vi "SOM.vi"(8 "Stopp":bool, 10 "SLOT":i32=100, 11 "USB":i32) -> ()   [LabVIEW 2020]
doc: "This VI provides a GUI for SOM modules. It implements an abstract module interface, where callers provide the only necessary and sufficient information for callee modules via the datafields USB, SLOT and Stopp. All module intern information are handled hidden by the module. Thereby, a caller must not \"know\" about such internals."
panel:
  in  "BurstDat[i]":T1={"[i]"=1, "BurstLen[i]"=1, "SyncEna[i]"=TRUE, "OutpEna[i]"=TRUE} {"BurstLen[i]" min=0 max=16777215 step=1}
  in  "Burst Data":T2(array[cluster]) {"BurstLen[i]" min=0 max=16777215 step=1}
  in  "AUX In Ctrl":u8(ring) items=["free running", "running if AUX IN is on High", "running if AUX IN is on Low"]
  in  "AUX Out Ctrl":u8(ring) items=["disabled", "enabled"]
  in  "Sync Enable":bool[](array[boolean])=[TRUE, FALSE, FALSE, TRUE, FALSE, FALSE, FALSE, FALSE]
  in  "Burst Out":bool[](array[boolean])=[TRUE, TRUE, FALSE, FALSE, TRUE, FALSE, FALSE, FALSE]
  in  "TriggerLevel [mV]":i32=421 min=-1200 max=1200 step=100 format="%5d"
  in  "Burst Length":i32[](array[numeric])=[1, 0, 2, 0, 0, 0, 0, 0]
  in  "Invert":bool=TRUE
  in  "Syncmask":u8
  in  "Presync":u8=4
  in  "Divider":u8=80
  in  "Base Osc./Trigger":i32(ring)=2
  # "Idx   Burst Length       Sync Enable       Out Enable"
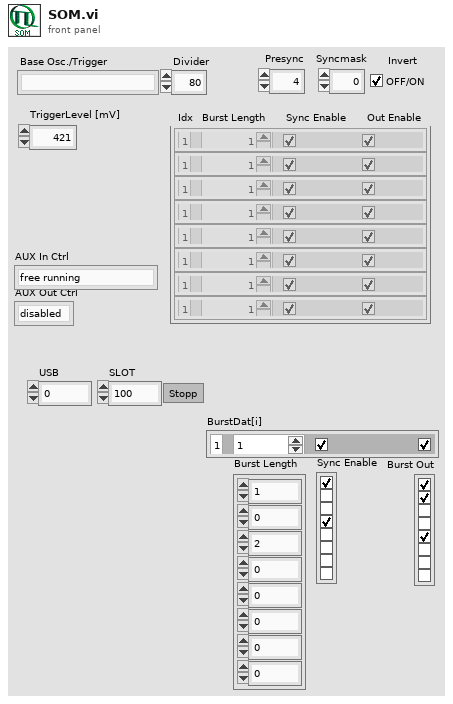
[diagram p1: front panel]
types:
  T1 = cluster{"[i]":i32, "BurstLen[i]":i32, "SyncEna[i]":bool, "OutpEna[i]":bool}
  T2 = cluster{"[i]":i32, "BurstLen[i]":i32, "SyncEna[i]":bool, "OutpEna[i]":bool}[]
  T3 = cluster{"Divider":u8, "PreSync":u8, "MaskSync":u8}
  T4 = cluster{"OutEnable":u8, "SyncEnable":u8, "SyncInverse":enum8{"Standard_Sync_Mask", "Inverse_Sync_Mask"}}
  T5 = cluster{"Divider":u8, "PreSync":u8, "SyncMask":u8}
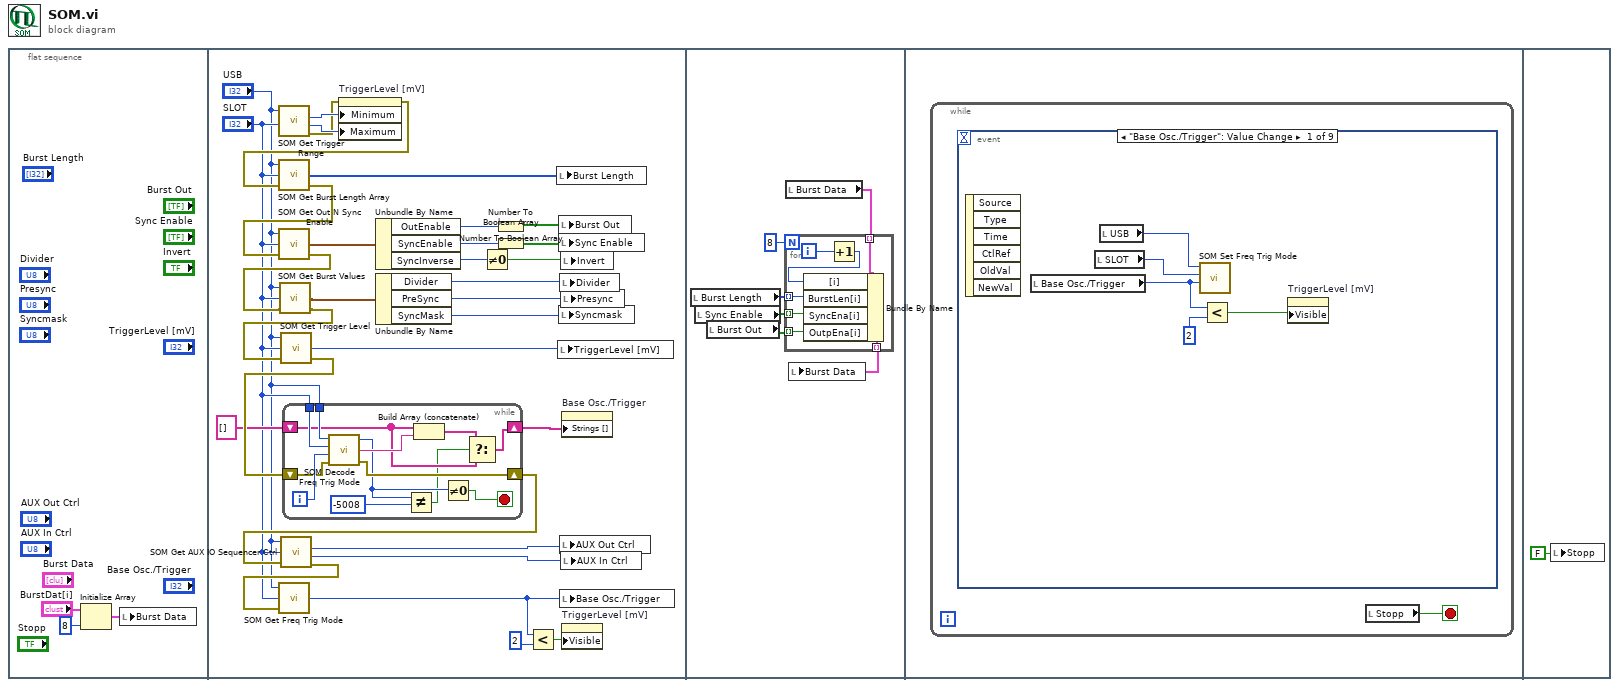
[diagram p0: block diagram]
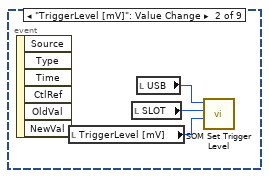
[diagram p2: hidden frame]
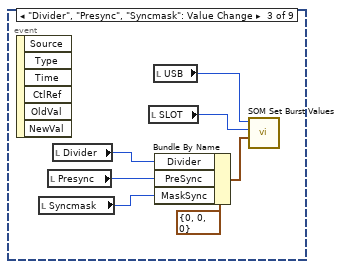
[diagram p3: hidden frame]
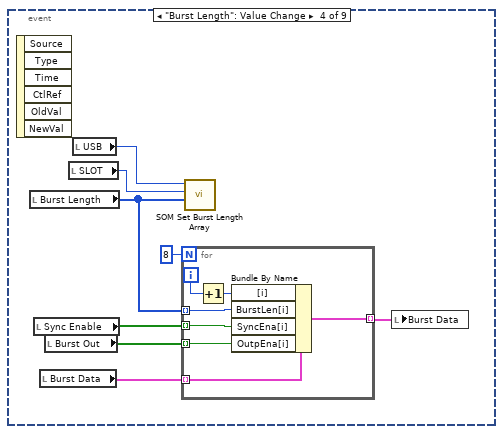
[diagram p4: hidden frame]
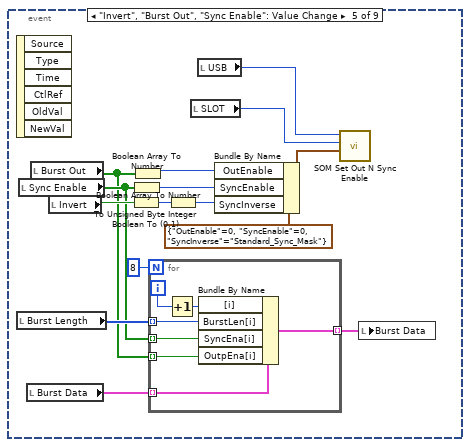
[diagram p5: hidden frame]
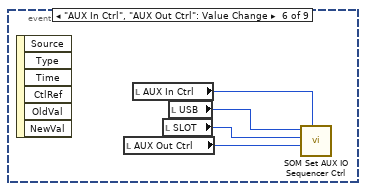
[diagram p6: hidden frame]
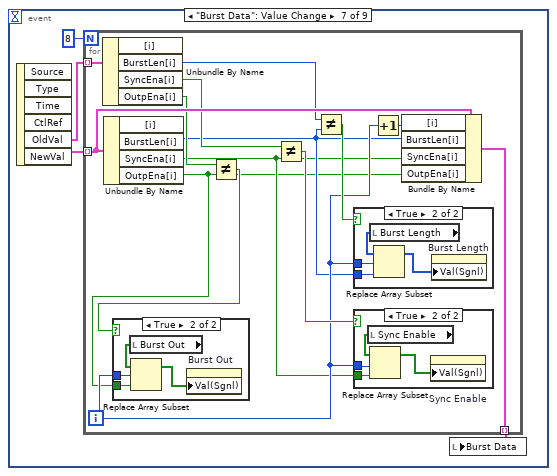
[diagram p7: hidden frame]
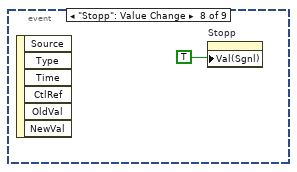
[diagram p11: hidden frame]
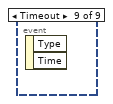
[diagram p12: hidden frame]
diagram:
  n1 = flat-sequence {
    frame #0 {
      n2 = Initialize Array("BurstDat[i]", 8 ("dimension size")) -> (w3:T2)
      n3 = local write "Burst Data"(w3) -> ()
    }
    frame #1 {
      n4 = call "SOM Get Trigger Range.vi"("DevIdx"="USB", "SlotId"="SLOT") -> ("MilliVoltLow"=w35:i32, "MilliVoltHigh"=w34:i32, "error out"=w33:errorcluster)  [unwired: 1 in, 1 out]
      n5 = property on="TriggerLevel [mV]" class="DigNum (strict)"(error in=w33, "Minimum"=w35, "Maximum"=w34) -> (error out=w32:errorcluster)  [unwired: 1 in, 1 out]
      n6 = call "SOM Get Burst Length Array.vi"("error in (no error)"=w32, "SlotId"="SLOT", "DevIdx"="USB") -> ("error out"=w12:errorcluster, "SOM Burst Length Array"=w5:i32[])  [unwired: 1 out]
      n7 = call "SOM Get Out N Sync Enable.vi"("error in (no error)"=w12, "SlotId"="SLOT", "DevIdx"="USB") -> ("error out"=w9:errorcluster, "SOM Out N Sync Enable"=w11:T4)  [unwired: 1 out]
      n8 = call "SOM Get Burst Values.vi"("error in (no error)"=w9, "SlotId"="SLOT", "DevIdx"="USB") -> ("error out"=w10:errorcluster, "SOM Burst Values"=w8:T5)  [unwired: 1 out]
      n9 = call "SOM Get Trigger Level.vi"("error in (no error)"=w10, "SlotId"="SLOT", "DevIdx"="USB") -> ("error out"=w21:errorcluster, "MilliVolt"=w22:i32)  [unwired: 1 out]
      n10 = while {
        tunnel: "USB" -> [w47]
        tunnel: "SLOT" -> [w46]
        shift-right: [w44] -> w15
        shift-left: w21 -> [w43]
        shift-right: [w39] -> w19
        shift-left: string[] [] -> [w37]
        i -> [w48]
        stop <- w45 stop-if-true
        n11 = call "SOM Decode Freq Trig Mode.vi"("error in (no error)"=w43, "FreqTrigMode"=w48, "SlotId"=w46, "DevIdx"=w47) -> ("error out"=w44:errorcluster, "FreqTrigMode"=w42:string, "function return"=w41:i32)
        n12 = Not Equal?(x=w41, y=-5008) -> (x != y?=w36:bool)
        n13 = Build Array (concatenate)(w37, w42) -> (w38:string[])
        n14 = Not Equal To 0?(x=w41) -> (x != 0?=w45:bool)
        n15 = Select(t=w38, s=w36, f=w37) -> (s? t:f=w39:string[])
      }
      n16 = call "SOM Get AUX IO Sequencer Ctrl.vi"("DevIdx"="USB", "SlotId"="SLOT", "error in (no error)"=w15) -> ("AUX Out Ctrl"=w4:u8, "AUX In Ctrl"=w13:u8, "error out"=w14:errorcluster)  [unwired: 1 out]
      n17 = call "SOM Get Freq Trig Mode.vi"("error in (no error)"=w14, "SlotId"="SLOT", "DevIdx"="USB") -> ("FreqTrigMode"=w16:i32)  [unwired: 2 out]
      n18 = Unbundle By Name(w11) -> ("OutEnable"=w31:u8, "SyncEnable"=w29:u8, "SyncInverse"=w27:enum8{"Standard_Sync_Mask", "Inverse_Sync_Mask"})
      n19 = Unbundle By Name(w8) -> ("Divider"=w23:u8, "PreSync"=w24:u8, "SyncMask"=w25:u8)
      n20 = Not Equal To 0?(x=w27) -> (x != 0?=w26:bool)
      n21 = Number To Boolean Array(number=w31) -> (Boolean array=w30:bool[])
      n22 = Number To Boolean Array(number=w29) -> (Boolean array=w28:bool[])
      n23 = Less?(x=w16, y=2) -> (x < y?=w18:bool)
      n24 = local write "Burst Length"(w5) -> ()
      n25 = local write "TriggerLevel [mV]"(w22) -> ()
      n26 = local write "Burst Out"(w30) -> ()
      n27 = local write "Sync Enable"(w28) -> ()
      n28 = local write "Syncmask"(w25) -> ()
      n29 = local write "Divider"(w23) -> ()
      n30 = local write "AUX Out Ctrl"(w4) -> ()
      n31 = local write "Base Osc./Trigger"(w16) -> ()
      n32 = local write "Invert"(w26) -> ()
      n33 = local write "Presync"(w24) -> ()
      n34 = local write "AUX In Ctrl"(w13) -> ()
      n35 = property on="Base Osc./Trigger" class="Ring (strict)"("Strings []"=w19) -> ()  [unwired: 2 in, 2 out]
      n36 = property on="TriggerLevel [mV]" class="DigNum (strict)"("Visible"=w18) -> ()  [unwired: 2 in, 2 out]
    }
    frame #2 {
      n37 = local read "Burst Length"() -> (w54:i32[])
      n38 = local read "Sync Enable"() -> (w53:bool[])
      n39 = local read "Burst Out"() -> (w52:bool[])
      n40 = local read "Burst Data"() -> (w50:T2)
      n41 = for {
        N: 8 -> [_]
        tunnel: w54 -> [w61] mode=indexing
        tunnel: w53 -> [w60] mode=indexing
        tunnel: w52 -> [w59] mode=indexing
        tunnel: w50 -> [w58] mode=indexing
        tunnel: [w55] -> w49 mode=indexing
        i -> [w56]
        n42 = Increment(x=w56) -> (x+1=w57:i32)
        n43 = Bundle By Name(cluster=w58, "[i]"=w57, "BurstLen[i]"=w61, "SyncEna[i]"=w60, "OutpEna[i]"=w59) -> (w55:T1)
      }
      n44 = local write "Burst Data"(w49) -> ()
    }
    frame #3 {
      n45 = while {
        stop <- w62 stop-if-true
        n46 = event shown="[0] \"Base Osc./Trigger\": Value Change" {
          selector: _ -> [_ _ _ _ _ _ _ _ _]
          dyn-events: _ -> [_ _ _ _ _ _ _ _ _]
          timeout: _ -> [_ _ _ _ _ _ _ _ _]
          event "Base Osc./Trigger": Value Change {
            n47 = event-data() -> ()  [unwired: 1 in, 6 out]
            n48 = local read "Base Osc./Trigger"() -> (w63:i32)
            n49 = local read "SLOT"() -> (w67:i32)
            n50 = local read "USB"() -> (w66:i32)
            n51 = call "SOM Set Freq Trig Mode.vi"("FreqTrigMode"=w63, "SlotId"=w67, "DevIdx"=w66) -> ()  [unwired: 1 in, 2 out]
            n52 = Less?(x=w63, y=2) -> (x < y?=w64:bool)
            n53 = property on="TriggerLevel [mV]" class="DigNum (strict)"("Visible"=w64) -> ()  [unwired: 2 in, 2 out]
          }
          event "TriggerLevel [mV]": Value Change {
            n54 = event-data() -> ()  [unwired: 1 in, 6 out]
            n55 = local read "TriggerLevel [mV]"() -> (w68:i32)
            n56 = local read "SLOT"() -> (w70:i32)
            n57 = local read "USB"() -> (w69:i32)
            n58 = call "SOM Set Trigger Level.vi"("MilliVolt"=w68, "SlotId"=w70, "DevIdx"=w69) -> ()  [unwired: 1 in, 2 out]
          }
          event "Divider", "Presync", "Syncmask": Value Change {
            n59 = event-data() -> ()  [unwired: 1 in, 6 out]
            n60 = local read "Syncmask"() -> (w71:u8)
            n61 = local read "Presync"() -> (w72:u8)
            n62 = local read "Divider"() -> (w73:u8)
            n63 = local read "SLOT"() -> (w77:i32)
            n64 = local read "USB"() -> (w76:i32)
            n65 = Bundle By Name(cluster=T3 {"Divider"=0, "PreSync"=0, "MaskSync"=0} ("SOM Burst Values"), "Divider"=w73, "PreSync"=w72, "MaskSync"=w71) -> (w74:T3)
            n66 = call "SOM Set Burst Values.vi"("SOM Burst Values"=w74, "SlotId"=w77, "DevIdx"=w76) -> ()  [unwired: 1 in, 2 out]
          }
          event "Burst Length": Value Change {
            n67 = event-data() -> ()  [unwired: 1 in, 6 out]
            n68 = local read "Burst Length"() -> (w80:i32[])
            n69 = local read "Sync Enable"() -> (w84:bool[])
            n70 = local read "Burst Data"() -> (w78:T2)
            n71 = local read "Burst Out"() -> (w83:bool[])
            n72 = local read "SLOT"() -> (w81:i32)
            n73 = local read "USB"() -> (w82:i32)
            n74 = for {
              N: 8 -> [_]
              tunnel: w80 -> [w92] mode=indexing
              tunnel: w84 -> [w91] mode=indexing
              tunnel: w83 -> [w90] mode=indexing
              tunnel: w78 -> [w89] mode=indexing
              tunnel: [w88] -> w85 mode=indexing
              i -> [w86]
              n75 = Increment(x=w86) -> (x+1=w87:i32)
              n76 = Bundle By Name(cluster=w89, "[i]"=w87, "BurstLen[i]"=w92, "SyncEna[i]"=w91, "OutpEna[i]"=w90) -> (w88:T1)
            }
            n77 = call "SOM Set Burst Length Array.vi"("SOM Burst Length Array"=w80, "SlotId"=w81, "DevIdx"=w82) -> ()  [unwired: 1 in, 2 out]
            n78 = local write "Burst Data"(w85) -> ()
          }
          event "Invert", "Burst Out", "Sync Enable": Value Change {
            n79 = event-data() -> ()  [unwired: 1 in, 6 out]
            n80 = local read "Burst Length"() -> (w102:i32[])
            n81 = local read "Sync Enable"() -> (w98:bool[])
            n82 = local read "Burst Data"() -> (w101:T2)
            n83 = local read "Burst Out"() -> (w96:bool[])
            n84 = local read "Invert"() -> (w104:bool)
            n85 = Boolean To (0,1)(Boolean=w104) -> (0, 1=w94:i16)
            n86 = Boolean Array To Number(Boolean array=w98) -> (number=w99:u8)
            n87 = Boolean Array To Number(Boolean array=w96) -> (number=w97:u8)
            n88 = for {
              N: 8 -> [_]
              tunnel: w102 -> [w114] mode=indexing
              tunnel: w98 -> [w113] mode=indexing
              tunnel: w96 -> [w112] mode=indexing
              tunnel: w101 -> [w111] mode=indexing
              tunnel: [w110] -> w100 mode=indexing
              i -> [w108]
              n89 = Increment(x=w108) -> (x+1=w109:i32)
              n90 = Bundle By Name(cluster=w111, "[i]"=w109, "BurstLen[i]"=w114, "SyncEna[i]"=w113, "OutpEna[i]"=w112) -> (w110:T1)
            }
            n91 = To Unsigned Byte Integer(number=w94) -> (unsigned 8bit integer=w95:u8)
            n92 = local read "SLOT"() -> (w107:i32)
            n93 = local read "USB"() -> (w106:i32)
            n94 = Bundle By Name(cluster=T4 {"OutEnable"=0, "SyncEnable"=0, "SyncInverse"=enum."Standard_Sync_Mask"} ("SOM Out N Sync Enable"), "OutEnable"=w97, "SyncEnable"=w99, "SyncInverse"=w95) -> (w103:T4)
            n95 = call "SOM Set Out N Sync Enable.vi"("SOM Out N Sync Enable"=w103, "SlotId"=w107, "DevIdx"=w106) -> ()  [unwired: 1 in, 2 out]
            n96 = local write "Burst Data"(w100) -> ()
          }
          event "AUX In Ctrl", "AUX Out Ctrl": Value Change {
            n97 = event-data() -> ()  [unwired: 1 in, 6 out]
            n98 = local read "AUX Out Ctrl"() -> (w118:u8)
            n99 = local read "AUX In Ctrl"() -> (w115:u8)
            n100 = local read "SLOT"() -> (w117:i32)
            n101 = local read "USB"() -> (w116:i32)
            n102 = call "SOM Set AUX IO Sequencer Ctrl.vi"("DevIdx"=w116, "SlotId"=w117, "AUX Out Ctrl"=w118, "AUX In Ctrl"=w115) -> ()  [unwired: 1 in, 2 out]
          }
          event "Burst Data": Value Change {
            n103 = event-data() -> ("OldVal"=w122:T2, "NewVal"=w121:T2)  [unwired: 1 in, 4 out]
            n104 = for {
              N: 8 -> [_]
              tunnel: w122 -> [w136] mode=indexing
              tunnel: w121 -> [w134] mode=indexing
              tunnel: [w135] -> w120 mode=indexing
              i -> [w126]
              n105 = Unbundle By Name(w136) -> ("BurstLen[i]"=w129:i32, "SyncEna[i]"=w132:bool, "OutpEna[i]"=w131:bool)  [unwired: 1 out]
              n106 = Unbundle By Name(w134) -> ("BurstLen[i]"=w125:i32, "SyncEna[i]"=w124:bool, "OutpEna[i]"=w123:bool)  [unwired: 1 out]
              n107 = Not Equal?(x=w131, y=w123) -> (x != y?=w127:bool)
              n108 = case shown="True" w127 {
                tunnel: w126 -> [_ w139]
                tunnel: w123 -> [_ w138]
                frame False {
                }
                frame True {
                  n109 = local read "Burst Out"() -> (w140:bool[])
                  n110 = Replace Array Subset(array=w140, new element=w138, index=w139) -> (w137:bool[])
                  n111 = property on="Burst Out" class="Arr (strict)"("Val(Sgnl)"=w137) -> ()  [unwired: 2 in, 2 out]
                }
              }
              n112 = Not Equal?(x=w132, y=w124) -> (x != y?=w128:bool)
              n113 = Not Equal?(x=w129, y=w125) -> (x != y?=w130:bool)
              n114 = case shown="True" w130 {
                tunnel: w126 -> [_ w147]
                tunnel: w125 -> [_ w146]
                frame False {
                }
                frame True {
                  n115 = local read "Burst Length"() -> (w148:i32[])
                  n116 = Replace Array Subset(array=w148, new element=w146, index=w147) -> (w145:i32[])
                  n117 = property on="Burst Length" class="Arr (strict)"("Val(Sgnl)"=w145) -> ()  [unwired: 2 in, 2 out]
                }
              }
              n118 = case shown="True" w128 {
                tunnel: w126 -> [_ w143]
                tunnel: w124 -> [_ w142]
                frame False {
                }
                frame True {
                  n119 = local read "Sync Enable"() -> (w144:bool[])
                  n120 = Replace Array Subset(array=w144, new element=w142, index=w143) -> (w141:bool[])
                  n121 = property on="Sync Enable" class="Arr (strict)"("Val(Sgnl)"=w141) -> ()  [unwired: 2 in, 2 out]
                }
              }
              n122 = Increment(x=w126) -> (x+1=w133:i32)
              n123 = Bundle By Name(cluster=w134, "[i]"=w133, "BurstLen[i]"=w125, "SyncEna[i]"=w124, "OutpEna[i]"=w123) -> (w135:T1)
            }
            n124 = local write "Burst Data"(w120) -> ()
          }
          event "Stopp": Value Change {
            n125 = event-data() -> ()  [unwired: 1 in, 6 out]
            n126 = property on="Stopp" class="Bool (strict)"("Val(Sgnl)"=TRUE ("Value (Signaling)")) -> ()  [unwired: 2 in, 2 out]
          }
          event Timeout {
            n127 = event-data() -> ()  [unwired: 1 in, 2 out]
          }
        }
        n128 = local read "Stopp"() -> (w62:bool)
      }
    }
    frame #4 {
      n129 = local write "Stopp"(FALSE ("Stopp")) -> ()
    }
  }
